vi "svx_Signal Generation (no HW).vi"(4 "noise amplitude":dbl=0.01 format="%.2f", 5 "pulse":T1={"square frequency"=20.0, "duty cycle (%)"=50.0} {"duty cycle (%)" format="%.2f"; "square frequency" format="%.2f"}, 6 "add noise (T)":bool=TRUE, 7 "pulsed (F)":bool, 8 "error in (no error)":errorcluster, 9 "window":T3(ring), 10 "df (dual tone)":dbl=100.0 format="%.2f", 11 "signal settings":T2={"signal type"=enum."Sine wave", "frequency"=1000.0, "amplitude"=1.0, "sampling info"={"sampling frequency"=51200.0, "#s"=4096.0}} {"sampling info"."#s" format="%.2f"; "sampling info"."sampling frequency" format="%.2p"; "amplitude" format="%.2f"; "frequency" format="%.2f"}) -> (0 "error out":errorcluster, 3 "signal out":waveform(dbl))   [LabVIEW 2017]
doc: "Simulates dynamic signals to demonstrate dynamic signal properties and Sound and Vibration measurement analyses."
uses:
  <vilib>/measure/macond.llb/Scaled Window for 1 Chan.vi
  <vilib>/measure/maUtilsandCtls.llb/ma_Updatet0 timestamp.vi
  <vilib>/addons/_NISVFA/_Generation/SoundVib_Generation.lvlib
  <vilib>/measure/NI_MABase.lvlib
  <vilib>/Analysis/NI_AALBase.lvlib
  <vilib>/measure/NI_MAPro.lvlib
panel:
  out "Waveform Graph":waveform(dbl)(graph)={"t0"=timestamp(0 s since 1904-01-01), "dt"=4.5351473922902495e-05, "Y"=[]}
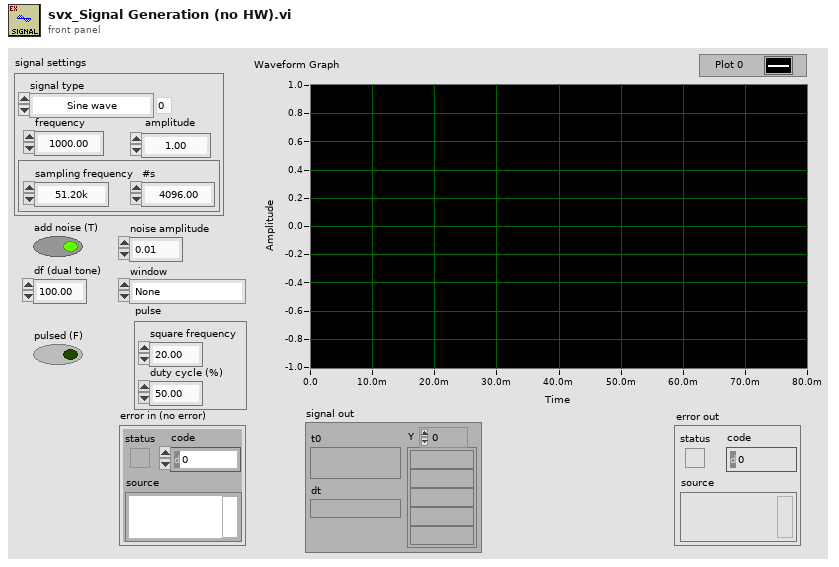
[diagram p1: front panel]
types:
  T1 = cluster{"square frequency":dbl, "duty cycle (%)":dbl}
  T2 = cluster{"signal type":enum16{"Sine wave", "Square wave", "Triangle wave", "Sawtooth wave", "Chirp", "Uniform white noise", "Gaussian white noise", "Pink noise", "PRN", "Dual tone"}, "frequency":dbl, "amplitude":dbl, "sampling info":cluster{"sampling frequency":dbl, "#s":dbl}}
  T3 = enum16{"None ", "Hanning", "Hamming", "Blackman-Harris", "Exact Blackman", "Blackman", "Flat Top", "4 Term B-Harris ", "7 Term B-Harris", "Low Sidelobe"}
  T4 = enum16{"Sine wave", "Square wave", "Triangle wave", "Sawtooth wave", "Chirp", "Uniform white noise", "Gaussian white noise", "Pink noise", "PRN", "Dual tone"}
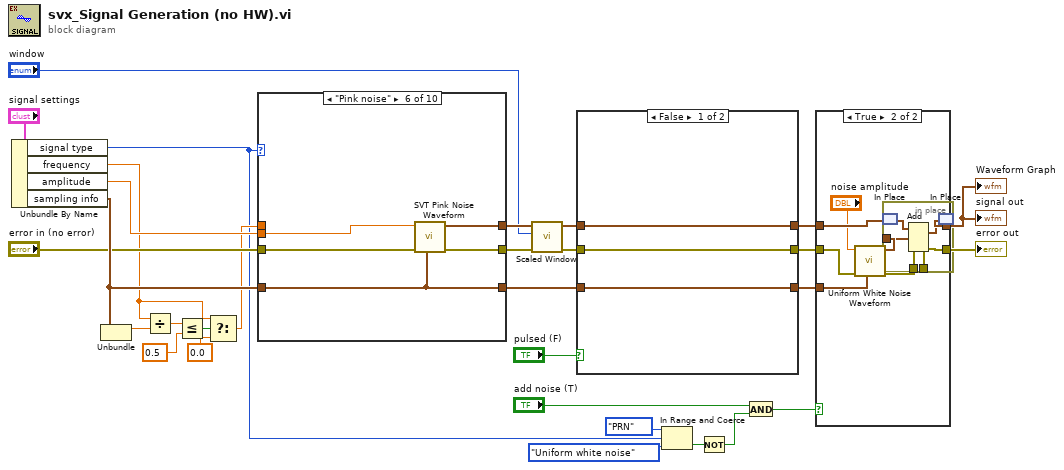
[diagram p0: block diagram]
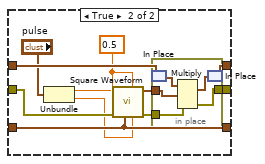
[diagram p2: hidden frame]
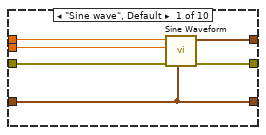
[diagram p4: hidden frame]
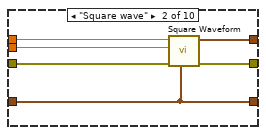
[diagram p5: hidden frame]
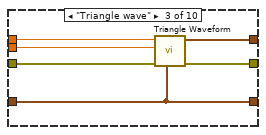
[diagram p6: hidden frame]
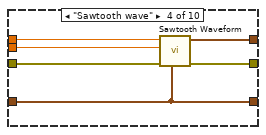
[diagram p7: hidden frame]
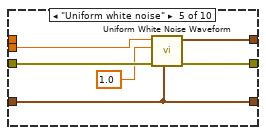
[diagram p8: hidden frame]
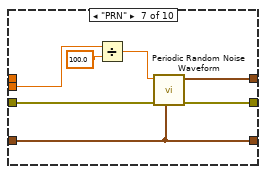
[diagram p9: hidden frame]
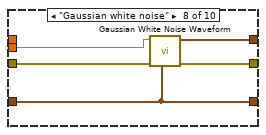
[diagram p10: hidden frame]
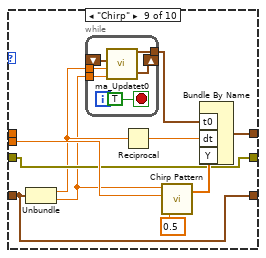
[diagram p11: hidden frame]
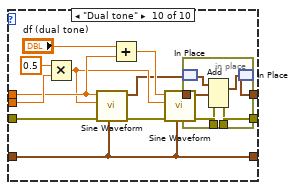
[diagram p12: hidden frame]
diagram:
  n1 = Unbundle By Name("signal settings") -> ("signal type"=w5:T4, "frequency"=w10:dbl, "amplitude"=w17:dbl, "sampling info"=w16:cluster{"sampling frequency":dbl, "#s":dbl})
  n2 = Unbundle(w16) -> ("sampling frequency"=w14:dbl)  [unwired: 1 out]
  n3 = Divide(x=w10, y=w14) -> (x/y=w13:dbl)
  n4 = Less Or Equal?(x=w13, y=0.5) -> (x <= y?=w11:bool)
  n5 = Select(t=w10, s=w11, f=0.0) -> (s? t:f=w9:dbl)
  n6 = case shown="\"Pink noise\"" w5 {
    tunnel: w17 -> [w35 w41 w47 w53 w60 w64 w68 w73 w86 w107]
    tunnel: w16 -> [w32 w38 w44 w50 w57 w62 w70 w75 w87 w94]
    tunnel: w9 -> [w36 w42 w48 w54 _ _ _ _ _ w102]
    tunnel: [w34 w40 w46 w52 w59 w65 w72 w76 w85 w98] -> w28
    tunnel: [w33 w39 w45 w51 w58 w63 w71 w77 w81 w95] -> w27
    tunnel: [w32 w38 w44 w50 w57 w62 w70 w75 w87 w94] -> w23
    tunnel: "error in (no error)" -> [w31 w37 w43 w49 w56 w61 w69 w74 w81 w104]
    frame "Sine wave", Default {
      n7 = call <vilib>:"Sine Waveform.vi"("sampling info"=w32, "error in (no error)"=w31, "amplitude"=w35, "frequency"=w36) -> ("error out"=w33:errorcluster, "signal out"=w34:waveform(dbl))  [unwired: 6 in]
    }
    frame "Square wave" {
      n8 = call <vilib>:"Square Waveform.vi"("sampling info"=w38, "error in (no error)"=w37, "amplitude"=w41, "frequency"=w42) -> ("error out"=w39:errorcluster, "signal out"=w40:waveform(dbl))  [unwired: 6 in]
    }
    frame "Triangle wave" {
      n9 = call <vilib>:"Triangle Waveform.vi"("sampling info"=w44, "error in (no error)"=w43, "amplitude"=w47, "frequency"=w48) -> ("error out"=w45:errorcluster, "signal out"=w46:waveform(dbl))  [unwired: 6 in]
    }
    frame "Sawtooth wave" {
      n10 = call <vilib>:"Sawtooth Waveform.vi"("sampling info"=w50, "error in (no error)"=w49, "amplitude"=w53, "frequency"=w54) -> ("error out"=w51:errorcluster, "signal out"=w52:waveform(dbl))  [unwired: 6 in]
    }
    frame "Uniform white noise" {
      n11 = call <vilib>:"Uniform White Noise Waveform.vi"("sampling info"=w57, "error in (no error)"=w56, "seed"=1.0, "amplitude"=w60) -> ("error out"=w58:errorcluster, "signal out"=w59:waveform(dbl))  [unwired: 6 in]
    }
    frame "Pink noise" {
      n12 = call <vilib>:"SVT Pink Noise Waveform.vi"("sampling info"=w62, "error in (no error)"=w61, "amplitude"=w64) -> ("error out"=w63:errorcluster, "pink noise signal"=w65:waveform(dbl))  [unwired: 7 in]
    }
    frame "PRN" {
      n13 = Divide(x=w68, y=100.0) -> (x/y=w67:dbl)
      n14 = call <vilib>:"Periodic Random Noise Waveform.vi"("sampling info"=w70, "error in (no error)"=w69, "spectral amplitude"=w67) -> ("error out"=w71:errorcluster, "signal out"=w72:waveform(dbl))  [unwired: 7 in]
    }
    frame "Gaussian white noise" {
      n15 = call <vilib>:"Gaussian White Noise Waveform.vi"("sampling info"=w75, "error in (no error)"=w74, "standard deviation"=w73) -> ("error out"=w77:errorcluster, "signal out"=w76:waveform(dbl))  [unwired: 7 in]
    }
    frame "Chirp" {
      n16 = Unbundle(w87) -> ("sampling frequency"=w80:dbl, "#s"=w79:dbl)
      n17 = while {
        shift-right: [w89] -> _
        shift-left: _ -> [w93]
        tunnel: w80 -> [w92]
        tunnel: w79 -> [w91]
        tunnel: [w88] -> w78
        stop <- TRUE stop-if-true
        n18 = call-poly <vilib>:"ma_Updatet0.vi"("samples"=w91, "sampling rate (S/s)"=w92, "tf previous"=w93) -> ("tf new"=w89:timestamp, "t0"=w88:timestamp)  [unwired: 1 in]
      }
      n19 = Reciprocal(x=w80) -> (1/x=w83:dbl)
      n20 = call <vilib>:"Chirp Pattern.vi"("f2"=0.5, "amplitude"=w86, "samples"=w79) -> ("Chirp Pattern"=w84:dbl[])  [unwired: 1 in, 1 out]
      n21 = Bundle By Name("t0"=w78, "dt"=w83, "Y"=w84) -> (w85:waveform(dbl))  [unwired: 1 in]
    }
    frame "Dual tone" {
      n22 = Multiply(x=0.5, y=w107) -> (x*y=w100:dbl)
      n23 = call <vilib>:"Sine Waveform.vi"("sampling info"=w94, "error in (no error)"=w104, "amplitude"=w100, "frequency"=w102) -> ("error out"=w103:errorcluster, "signal out"=w97:waveform(dbl))  [unwired: 6 in]
      n24 = Add(x="df (dual tone)", y=w102) -> (x+y=w101:dbl)
      n25 = call <vilib>:"Sine Waveform.vi"("sampling info"=w94, "error in (no error)"=w103, "amplitude"=w100, "frequency"=w101) -> ("error out"=w96:errorcluster, "signal out"=w99:waveform(dbl))  [unwired: 6 in]
      n26 = in-place {
        in-place-border: w99 -> [w112]
        in-place-border: w96 -> [w109]
        in-place-border: [w108] -> w95
        n27 = in-place-match #1(w97) -> (w110:waveform(dbl))
        n28 = Add(1:w112, 2:w110, 4:w109) -> (0:w111:waveform(dbl), 3:w108:errorcluster)
        n29 = in-place-match #1(w111) -> (w98:waveform(dbl))
      }
    }
  }
  n30 = call-poly <vilib>:"Scaled Window.vi"("error in (no error)"=w27, "window"="window", "signal in"=w28) -> ("error out"=w24:errorcluster, "signal out"=w25:waveform(dbl))  [unwired: 6 in, 1 out]
  n31 = case shown="False" "pulsed (F)" {
    tunnel: w25 -> [w115 w126]
    tunnel: w24 -> [w114 w123]
    tunnel: w23 -> [w113 w119]
    tunnel: [w114 w122] -> w22
    tunnel: [w115 w121] -> w21
    tunnel: [w113 w119] -> w20
    frame False {
    }
    frame True {
      w120 = 0.5 ("amplitude")
      n32 = Unbundle("pulse") -> ("square frequency"=w117:dbl, "duty cycle (%)"=w116:dbl)
      n33 = call <vilib>:"Square Waveform.vi"("duty cycle (%)"=w116, "offset"=w120, "sampling info"=w119, "error in (no error)"=w123, "amplitude"=w120, "frequency"=w117) -> ("error out"=w124:errorcluster, "signal out"=w125:waveform(dbl))  [unwired: 4 in]
      n34 = in-place {
        in-place-border: w125 -> [w130]
        in-place-border: w124 -> [w129]
        in-place-border: [w128] -> w122
        n35 = in-place-match #2(w126) -> (w131:waveform(dbl))
        n36 = Multiply(1:w130, 2:w131, 4:w129) -> (0:w127:waveform(dbl), 3:w128:errorcluster)
        n37 = in-place-match #2(w127) -> (w121:waveform(dbl))
      }
    }
  }
  n38 = In Range and Coerce(upper limit=T4."PRN", x=w5, lower limit=T4."Uniform white noise") -> (In Range?=w6:bool)  [unwired: 1 out]
  n39 = Not(x=w6) -> (.not. x?=w1:bool)
  n40 = And(x="add noise (T)", y=w1) -> (x .and. y?=w7:bool)
  n41 = case shown="True" w7 {
    tunnel: w20 -> [_ w141]
    tunnel: w21 -> [w133 w140]
    tunnel: [w132 w138] -> w30
    tunnel: [w133 w137] -> w29
    tunnel: w22 -> [w132 w134]
    frame False {
    }
    frame True {
      n42 = call <vilib>:"Uniform White Noise Waveform.vi"("sampling info"=w141, "error in (no error)"=w134, "amplitude"="noise amplitude") -> ("error out"=w139:errorcluster, "signal out"=w136:waveform(dbl))  [unwired: 7 in]
      n43 = in-place {
        in-place-border: w139 -> [w145]
        in-place-border: [w144] -> w138
        in-place-border: w136 -> [w142]
        n44 = in-place-match #3(w140) -> (w146:waveform(dbl))
        n45 = Add(1:w142, 2:w146, 4:w145) -> (0:w143:waveform(dbl), 3:w144:errorcluster)
        n46 = in-place-match #3(w143) -> (w137:waveform(dbl))
      }
    }
  }
  "signal out" <- w29
  "error out" <- w30
  "Waveform Graph" <- w29
